vi "_Clear.vi"(6 "Variant in":variant, 8 "error in (no error)":errorcluster, 9 "Shift Pressed?":bool, 10 "QD Combo Box Ref":refnum<vi>, 11 "QD Launch VI Ref":refnum<vi>) -> (0 "error out":errorcluster, 4 "Variant out":variant)   [LabVIEW 2014, in "NEVSTOP QD Shortcuts.lvlib"]
uses:
  NEVSTOP QD Shortcuts.lvlib
panel:
  # "Do not change the connector pane of this VI.\n\nSee the block diagram for directions on how to use this template."
  # "Specify the name of the Undo transaction"
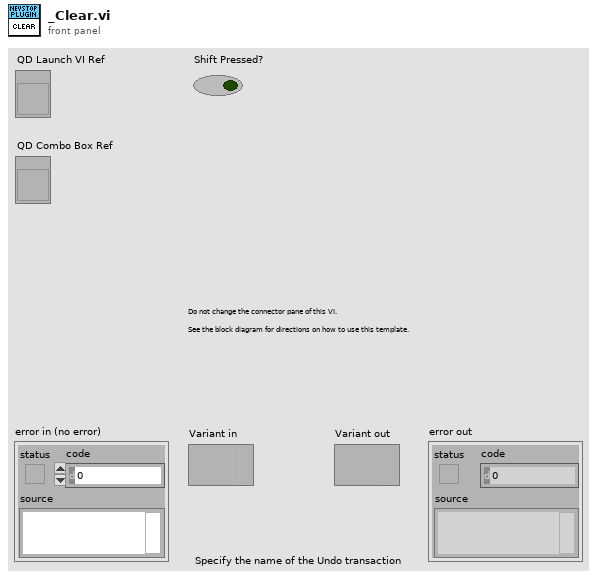
[diagram p1: front panel]
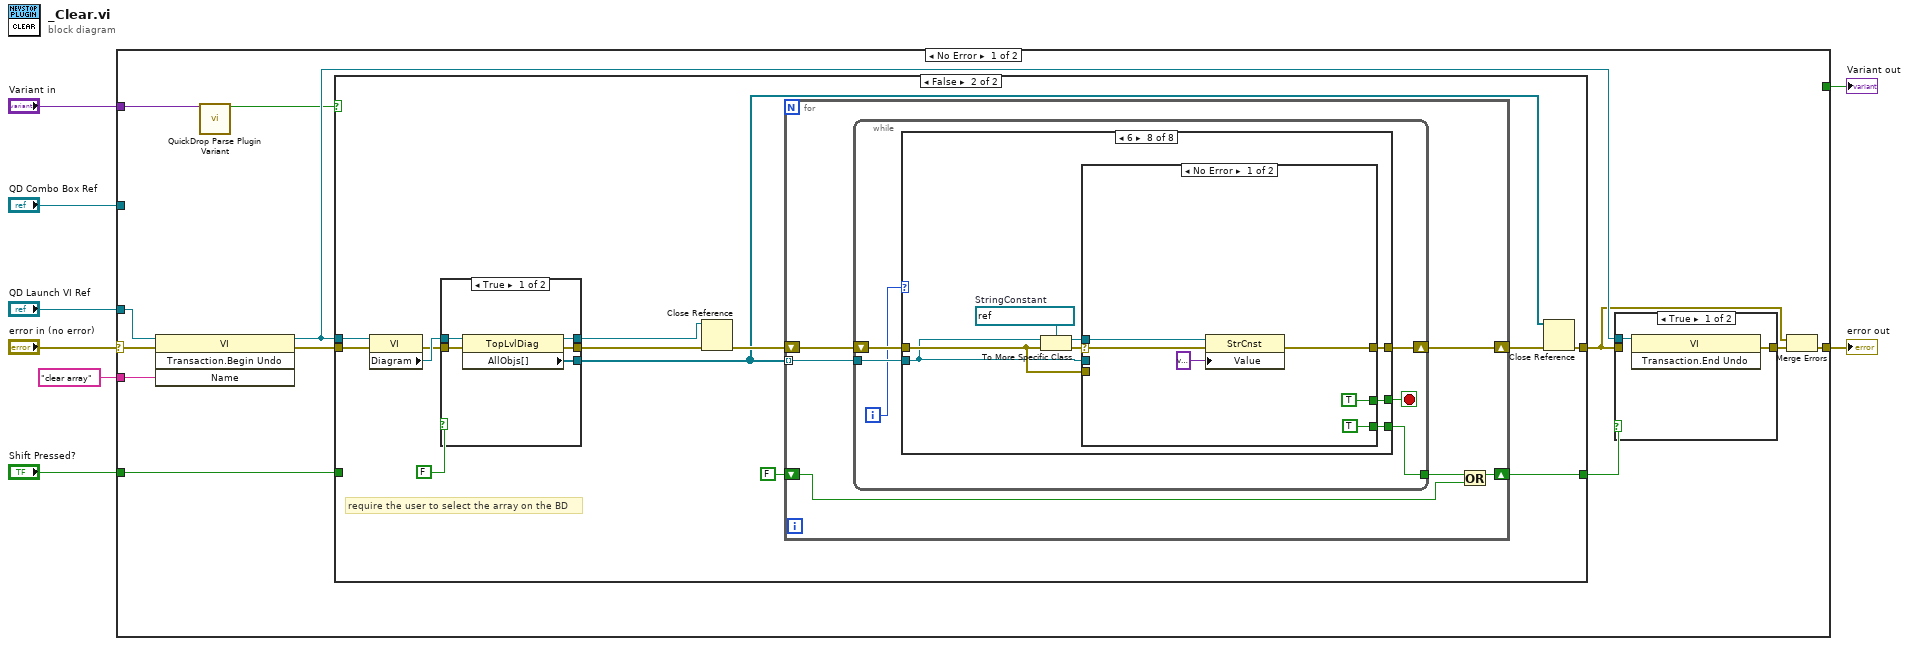
[diagram p0: block diagram]
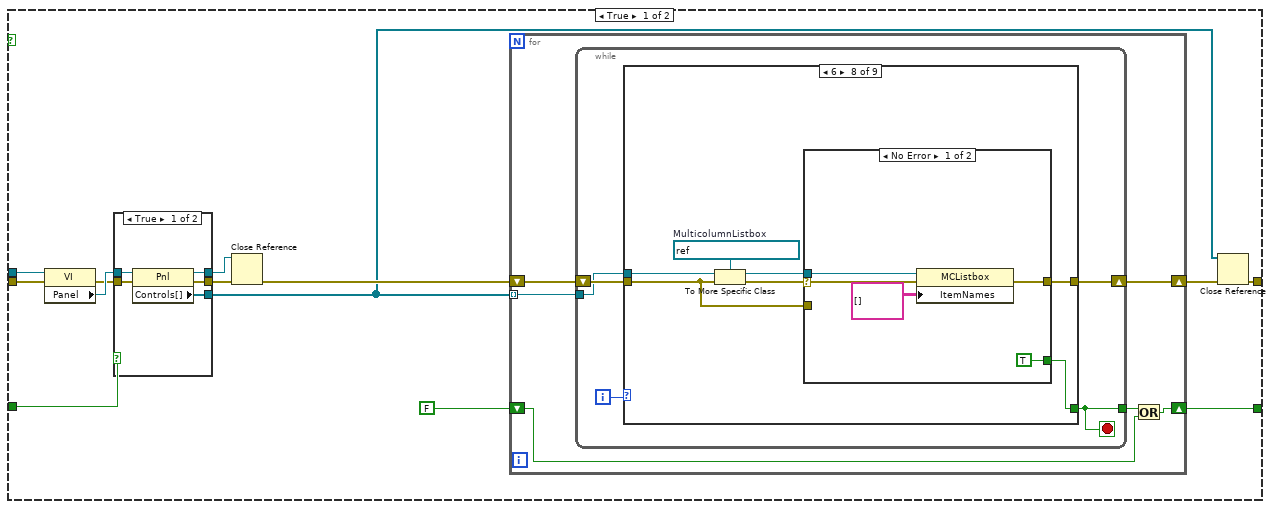
[diagram p2: hidden frame]
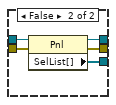
[diagram p3: hidden frame]
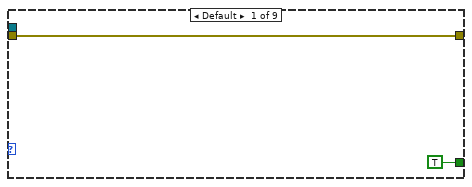
[diagram p4: hidden frame]
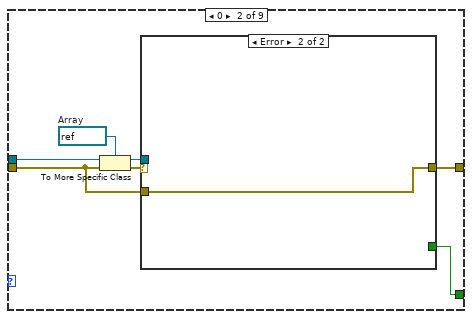
[diagram p5: hidden frame]
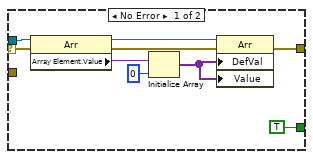
[diagram p6: hidden frame]
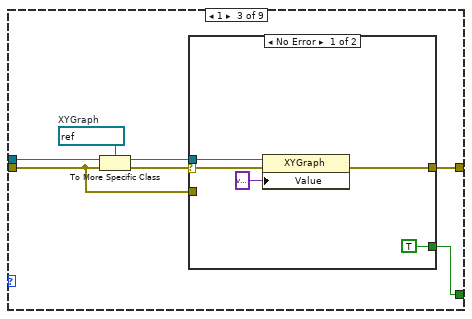
[diagram p7: hidden frame]
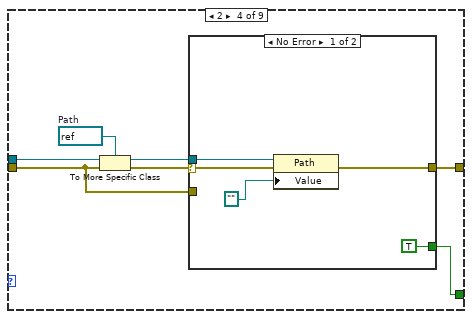
[diagram p9: hidden frame]
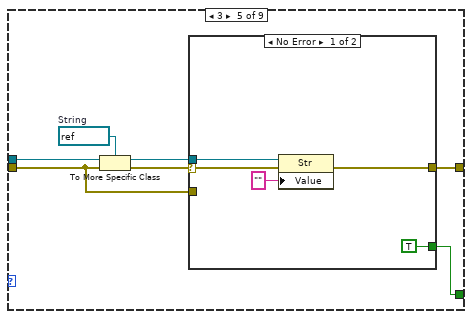
[diagram p11: hidden frame]
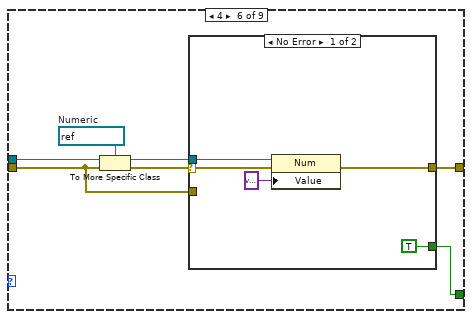
[diagram p13: hidden frame]
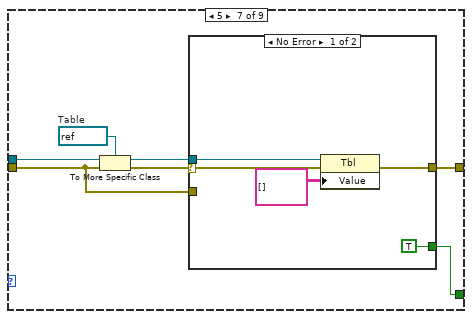
[diagram p15: hidden frame]
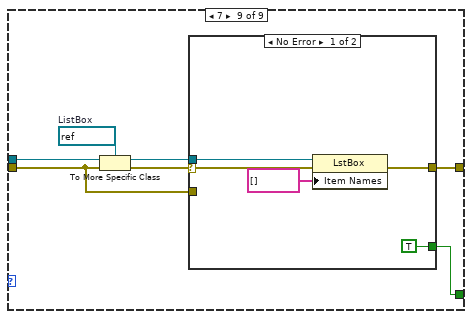
[diagram p18: hidden frame]
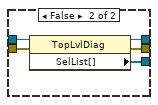
[diagram p20: hidden frame]
diagram:
  n1 = case shown="No Error" "error in (no error)" {
    selector: "error in (no error)" -> [w20 w316]
    tunnel: [w10 w316] -> w7
    tunnel: "QD Launch VI Ref" -> [w19 _]
    tunnel: "Shift Pressed?" -> [w14 _]
    tunnel: "QD Combo Box Ref" -> [_ _]
    tunnel: "Variant in" -> [w21 _]
    tunnel: "clear array" ("Undo Name") -> [w18 _]
    tunnel: [TRUE _] -> w1
    frame No Error {
      n2 = invoke class="VI" method="Transaction.Begin Undo"(reference=w19, error in=w20, "Name"=w18) -> (reference out=w13:refnum<vi>, error out=w16:errorcluster)  [unwired: 1 in, 2 out]
      n3 = call <vilib>:"QuickDrop Parse Plugin Variant.vi"("QDKS Variant in"=w21) -> ("QD Launch VI Panel?"=w12:bool)  [unwired: 12 in, 2 out]
      n4 = case shown="False" w12 {
        tunnel: w16 -> [w34 w178]
        tunnel: [w30 w175] -> w9
        tunnel: w14 -> [w25 _]
        tunnel: w13 -> [w28 w173]
        tunnel: [w23 w169] -> w11
        frame True {
          n5 = property class="VI"(reference=w28, error in=w34) -> (error out=w26:errorcluster, "Panel"=w27:refnum<vi>)  [unwired: 1 out]
          n6 = case shown="True" w25 {
            tunnel: [w39 w44] -> w32
            tunnel: [w38 w43] -> w31
            tunnel: [w37 w42] -> w29
            tunnel: w27 -> [w36 w41]
            tunnel: w26 -> [w35 w40]
            frame True {
              n7 = property class="Pnl"(reference=w36, error in=w35) -> (reference out=w38:refnum<vi>, error out=w39:errorcluster, "Controls[]"=w37:refnum<vi>[])
            }
            frame False {
              n8 = property class="Pnl"(reference=w41, error in=w40) -> (reference out=w43:refnum<vi>, error out=w44:errorcluster, "SelList[]"=w42:refnum<vi>[])
            }
          }
          n9 = Close Reference(reference=w31, error in (no error)=w32) -> (error out=w33:errorcluster)
          n10 = for {
            shift-right: [w50] -> w24
            shift-left: w33 -> [w49]
            tunnel: w29 -> [w48] mode=indexing
            shift-right: [w46] -> w23
            shift-left: FALSE -> [w45]
            n11 = while {
              tunnel: w48 -> [w53]
              tunnel: [w52] -> w47
              shift-right: [w55] -> w50
              shift-left: w49 -> [w54]
              i -> [w51]
              stop <- w52 stop-if-true
              n12 = case shown="6" w51 {
                tunnel: [w57 w64 w81 w94 w107 w120 w133 w146 w159] -> w55
                tunnel: w54 -> [w57 w61 w78 w91 w104 w117 w130 w143 w156]
                tunnel: w53 -> [_ w60 w77 w90 w103 w116 w129 w142 w155]
                tunnel: [TRUE w58 w75 w88 w101 w114 w127 w140 w153] -> w52
                frame Default {
                }
                frame 0 {
                  w59 = refnum<vi> refnum  # Array
                  n13 = To More Specific Class(target class=w59, reference=w60, error in=w61) -> (specific class reference=w63:refnum<vi>, error out=w62:errorcluster)
                  n14 = case shown="Error" w62 {
                    selector: w62 -> [w68 _]
                    tunnel: [w67 w74] -> w64
                    tunnel: w63 -> [w69 _]
                    tunnel: w61 -> [_ w74]
                    tunnel: [TRUE _] -> w58
                    frame No Error {
                      n15 = property class="Arr"(reference=w69, error in=w68) -> (reference out=w72:refnum<vi>, error out=w73:errorcluster, "Array Element.Value"=w71:variant)
                      n16 = Initialize Array(w71, 0 ("dimension size")) -> (w66:variant[])
                      n17 = property class="Arr"(reference=w72, error in=w73, "DefVal"=w66, "Value"=w66) -> (error out=w67:errorcluster)  [unwired: 1 out]
                    }
                    frame Error {
                    }
                  }
                }
                frame 1 {
                  w76 = refnum<vi> refnum  # XYGraph
                  n18 = To More Specific Class(target class=w76, reference=w77, error in=w78) -> (specific class reference=w80:refnum<vi>, error out=w79:errorcluster)
                  n19 = case shown="No Error" w79 {
                    selector: w79 -> [w86 _]
                    tunnel: [w84 w87] -> w81
                    tunnel: w80 -> [w85 _]
                    tunnel: w78 -> [_ w87]
                    tunnel: [TRUE _] -> w75
                    frame No Error {
                      n20 = property class="XYGraph"(reference=w85, error in=w86, "Value"=variant) -> (error out=w84:errorcluster)  [unwired: 1 out]
                    }
                    frame Error {
                    }
                  }
                }
                frame 2 {
                  w89 = refnum<vi> refnum  # Path
                  n21 = To More Specific Class(target class=w89, reference=w90, error in=w91) -> (specific class reference=w93:refnum<vi>, error out=w92:errorcluster)
                  n22 = case shown="No Error" w92 {
                    selector: w92 -> [w99 _]
                    tunnel: [w97 w100] -> w94
                    tunnel: w93 -> [w98 _]
                    tunnel: w91 -> [_ w100]
                    tunnel: [TRUE _] -> w88
                    frame No Error {
                      n23 = property class="Path"(reference=w98, error in=w99, "Value"=path "") -> (error out=w97:errorcluster)  [unwired: 1 out]
                    }
                    frame Error {
                    }
                  }
                }
                frame 3 {
                  w102 = refnum<vi> refnum  # String
                  n24 = To More Specific Class(target class=w102, reference=w103, error in=w104) -> (specific class reference=w106:refnum<vi>, error out=w105:errorcluster)
                  n25 = case shown="No Error" w105 {
                    selector: w105 -> [w112 _]
                    tunnel: [w110 w113] -> w107
                    tunnel: w106 -> [w111 _]
                    tunnel: w104 -> [_ w113]
                    tunnel: [TRUE _] -> w101
                    frame No Error {
                      n26 = property class="Str"(reference=w111, error in=w112, "Value"="") -> (error out=w110:errorcluster)  [unwired: 1 out]
                    }
                    frame Error {
                    }
                  }
                }
                frame 4 {
                  w115 = refnum<vi> refnum  # Numeric
                  n27 = To More Specific Class(target class=w115, reference=w116, error in=w117) -> (specific class reference=w119:refnum<vi>, error out=w118:errorcluster)
                  n28 = case shown="No Error" w118 {
                    selector: w118 -> [w125 _]
                    tunnel: [w123 w126] -> w120
                    tunnel: w119 -> [w124 _]
                    tunnel: w117 -> [_ w126]
                    tunnel: [TRUE _] -> w114
                    frame No Error {
                      n29 = property class="Num"(reference=w124, error in=w125, "Value"=variant) -> (error out=w123:errorcluster)  [unwired: 1 out]
                    }
                    frame Error {
                    }
                  }
                }
                frame 5 {
                  w128 = refnum<vi> refnum  # Table
                  n30 = To More Specific Class(target class=w128, reference=w129, error in=w130) -> (specific class reference=w132:refnum<vi>, error out=w131:errorcluster)
                  n31 = case shown="No Error" w131 {
                    selector: w131 -> [w138 _]
                    tunnel: [w136 w139] -> w133
                    tunnel: w132 -> [w137 _]
                    tunnel: w130 -> [_ w139]
                    tunnel: [TRUE _] -> w127
                    frame No Error {
                      n32 = property class="Tbl"(reference=w137, error in=w138, "Value"=string[][] []) -> (error out=w136:errorcluster)  [unwired: 1 out]
                    }
                    frame Error {
                    }
                  }
                }
                frame 6 {
                  w141 = refnum<vi> refnum  # MulticolumnListbox
                  n33 = To More Specific Class(target class=w141, reference=w142, error in=w143) -> (specific class reference=w145:refnum<vi>, error out=w144:errorcluster)
                  n34 = case shown="No Error" w144 {
                    selector: w144 -> [w151 _]
                    tunnel: [w149 w152] -> w146
                    tunnel: w145 -> [w150 _]
                    tunnel: w143 -> [_ w152]
                    tunnel: [TRUE _] -> w140
                    frame No Error {
                      n35 = property class="MCListbox"(reference=w150, error in=w151, "ItemNames"=string[][] [] ("Item Names")) -> (error out=w149:errorcluster)  [unwired: 1 out]
                    }
                    frame Error {
                    }
                  }
                }
                frame 7 {
                  w154 = refnum<vi> refnum  # ListBox
                  n36 = To More Specific Class(target class=w154, reference=w155, error in=w156) -> (specific class reference=w158:refnum<vi>, error out=w157:errorcluster)
                  n37 = case shown="No Error" w157 {
                    selector: w157 -> [w164 _]
                    tunnel: [w162 w165] -> w159
                    tunnel: w158 -> [w163 _]
                    tunnel: w156 -> [_ w165]
                    tunnel: [TRUE _] -> w153
                    frame No Error {
                      n38 = property class="LstBox"(reference=w163, error in=w164, "Item Names"=string[] []) -> (error out=w162:errorcluster)  [unwired: 1 out]
                    }
                    frame Error {
                    }
                  }
                }
              }
            }
            n39 = Or(x=w47, y=w45) -> (x .or. y?=w46:bool)
          }
          n40 = Close Reference(reference=w29, error in (no error)=w24) -> (error out=w30:errorcluster)
        }
        frame False {
          # "require the user to select the array on the BD"
          n41 = property class="VI"(reference=w173, error in=w178) -> (error out=w171:errorcluster, "Diagram"=w172:refnum<vi>)  [unwired: 1 out]
          n42 = case shown="True" FALSE {
            tunnel: [w183 w188] -> w176
            tunnel: [w182 w187] -> w166
            tunnel: [w181 w186] -> w174
            tunnel: w172 -> [w180 w185]
            tunnel: w171 -> [w179 w184]
            frame True {
              n43 = property class="TopLvlDiag"(reference=w180, error in=w179) -> (reference out=w182:refnum<vi>, error out=w183:errorcluster, "AllObjs[]"=w181:refnum<vi>[])
            }
            frame False {
              n44 = property class="TopLvlDiag"(reference=w185, error in=w184) -> (reference out=w187:refnum<vi>, error out=w188:errorcluster, "SelList[]"=w186:refnum<vi>[])
            }
          }
          n45 = Close Reference(reference=w166, error in (no error)=w176) -> (error out=w177:errorcluster)
          n46 = for {
            shift-right: [w194] -> w170
            shift-left: w177 -> [w193]
            tunnel: w174 -> [w189] mode=indexing
            shift-right: [w191] -> w169
            shift-left: FALSE -> [w190]
            n47 = while {
              tunnel: [w198] -> w192
              tunnel: w189 -> [w197]
              shift-right: [w200] -> w194
              shift-left: w193 -> [w199]
              i -> [w196]
              stop <- w195 stop-if-true
              n48 = case shown="6" w196 {
                tunnel: [w202 w210 w229 w244 w259 w274 w289 w304] -> w200
                tunnel: w199 -> [w202 w207 w226 w241 w256 w271 w286 w301]
                tunnel: [_ w205 w224 w239 w254 w269 w284 w299] -> w198
                tunnel: w197 -> [_ w204 w223 w238 w253 w268 w283 w298]
                tunnel: [TRUE w203 w222 w237 w252 w267 w282 w297] -> w195
                frame Default {
                }
                frame 0 {
                  w206 = refnum<vi> refnum  # ArrayConstant
                  n49 = To More Specific Class(target class=w206, reference=w204, error in=w207) -> (specific class reference=w209:refnum<vi>, error out=w208:errorcluster)
                  n50 = case shown="No Error" w208 {
                    selector: w208 -> [w215 _]
                    tunnel: [w214 w221] -> w210
                    tunnel: w209 -> [w216 _]
                    tunnel: w207 -> [_ w221]
                    tunnel: [TRUE _] -> w205
                    tunnel: w204 -> [_ _]
                    tunnel: [TRUE _] -> w203
                    frame No Error {
                      n51 = property class="ArrCnst"(reference=w216, error in=w215) -> (reference out=w219:refnum<vi>, error out=w220:errorcluster, "Element.Value"=w218:variant)
                      n52 = Initialize Array(w218, 0 ("dimension size")) -> (w212:variant[])
                      n53 = property class="ArrCnst"(reference=w219, error in=w220, "Value"=w212) -> (error out=w214:errorcluster)  [unwired: 1 out]
                    }
                    frame Error {
                    }
                  }
                }
                frame 1 {
                  w225 = refnum<vi> refnum  # NumericConstant
                  n54 = To More Specific Class(target class=w225, reference=w223, error in=w226) -> (specific class reference=w228:refnum<vi>, error out=w227:errorcluster)
                  n55 = case shown="No Error" w227 {
                    selector: w227 -> [w235 _]
                    tunnel: [w233 w236] -> w229
                    tunnel: w228 -> [w234 _]
                    tunnel: w226 -> [_ w236]
                    tunnel: [TRUE _] -> w224
                    tunnel: w223 -> [_ _]
                    tunnel: [TRUE _] -> w222
                    frame No Error {
                      n56 = property class="NumericConstant"(reference=w234, error in=w235, "Value"=variant) -> (error out=w233:errorcluster)  [unwired: 1 out]
                    }
                    frame Error {
                    }
                  }
                }
                frame 2 {
                  w240 = refnum<vi> refnum  # Table
                  n57 = To More Specific Class(target class=w240, reference=w238, error in=w241) -> (specific class reference=w243:refnum<vi>, error out=w242:errorcluster)
                  n58 = case shown="No Error" w242 {
                    selector: w242 -> [w250 _]
                    tunnel: [w248 w251] -> w244
                    tunnel: w243 -> [w249 _]
                    tunnel: w241 -> [_ w251]
                    tunnel: [TRUE _] -> w239
                    tunnel: w238 -> [_ _]
                    tunnel: [TRUE _] -> w237
                    frame No Error {
                      n59 = property class="Tbl"(reference=w249, error in=w250, "Value"=string[][] []) -> (error out=w248:errorcluster)  [unwired: 1 out]
                    }
                    frame Error {
                    }
                  }
                }
                frame 3 {
                  w255 = refnum<vi> refnum  # MulticolumnListbox
                  n60 = To More Specific Class(target class=w255, reference=w253, error in=w256) -> (specific class reference=w258:refnum<vi>, error out=w257:errorcluster)
                  n61 = case shown="No Error" w257 {
                    selector: w257 -> [w265 _]
                    tunnel: [w263 w266] -> w259
                    tunnel: w258 -> [w264 _]
                    tunnel: w256 -> [_ w266]
                    tunnel: [TRUE _] -> w254
                    tunnel: w253 -> [_ _]
                    tunnel: [TRUE _] -> w252
                    frame No Error {
                      n62 = property class="MCListbox"(reference=w264, error in=w265, "ItemNames"=string[][] [] ("Item Names")) -> (error out=w263:errorcluster)  [unwired: 1 out]
                    }
                    frame Error {
                    }
                  }
                }
                frame 4 {
                  w270 = refnum<vi> refnum  # ListBox
                  n63 = To More Specific Class(target class=w270, reference=w268, error in=w271) -> (specific class reference=w273:refnum<vi>, error out=w272:errorcluster)
                  n64 = case shown="No Error" w272 {
                    selector: w272 -> [w280 _]
                    tunnel: [w278 w281] -> w274
                    tunnel: w273 -> [w279 _]
                    tunnel: w271 -> [_ w281]
                    tunnel: [TRUE _] -> w269
                    tunnel: w268 -> [_ _]
                    tunnel: [TRUE _] -> w267
                    frame No Error {
                      n65 = property class="LstBox"(reference=w279, error in=w280, "Item Names"=string[] []) -> (error out=w278:errorcluster)  [unwired: 1 out]
                    }
                    frame Error {
                    }
                  }
                }
                frame 5 {
                  w285 = refnum<vi> refnum  # PathConstant
                  n66 = To More Specific Class(target class=w285, reference=w283, error in=w286) -> (specific class reference=w288:refnum<vi>, error out=w287:errorcluster)
                  n67 = case shown="No Error" w287 {
                    selector: w287 -> [w295 _]
                    tunnel: [w293 w296] -> w289
                    tunnel: w288 -> [w294 _]
                    tunnel: w286 -> [_ w296]
                    tunnel: [TRUE _] -> w284
                    tunnel: w283 -> [_ _]
                    tunnel: [TRUE _] -> w282
                    frame No Error {
                      n68 = property class="PthCnst"(reference=w294, error in=w295, "Value"=variant) -> (error out=w293:errorcluster)  [unwired: 1 out]
                    }
                    frame Error {
                    }
                  }
                }
                frame 6 {
                  w300 = refnum<vi> refnum  # StringConstant
                  n69 = To More Specific Class(target class=w300, reference=w298, error in=w301) -> (specific class reference=w303:refnum<vi>, error out=w302:errorcluster)
                  n70 = case shown="No Error" w302 {
                    selector: w302 -> [w310 _]
                    tunnel: [w308 w311] -> w304
                    tunnel: w303 -> [w309 _]
                    tunnel: w301 -> [_ w311]
                    tunnel: [TRUE _] -> w299
                    tunnel: w298 -> [_ _]
                    tunnel: [TRUE _] -> w297
                    frame No Error {
                      n71 = property class="StrCnst"(reference=w309, error in=w310, "Value"=variant) -> (error out=w308:errorcluster)  [unwired: 1 out]
                    }
                    frame Error {
                    }
                  }
                }
              }
            }
            n72 = Or(x=w192, y=w190) -> (x .or. y?=w191:bool)
          }
          n73 = Close Reference(reference=w174, error in (no error)=w170) -> (error out=w175:errorcluster)
        }
      }
      n74 = case shown="True" w11 {
        tunnel: w13 -> [w312 w314]
        tunnel: [w313 w315] -> w15
        tunnel: w9 -> [_ _]
        frame True {
          n75 = invoke class="VI" method="Transaction.End Undo"(reference=w312) -> (error out=w313:errorcluster)  [unwired: 2 in, 2 out]
        }
        frame False {
          n76 = invoke class="VI" method="Transaction.Fail"(reference=w314) -> (error out=w315:errorcluster)  [unwired: 2 in, 2 out]
        }
      }
      n77 = Merge Errors(w9, w15) -> (w10:errorcluster)
    }
    frame Error {
    }
  }
  "error out" <- w7
  "Variant out" <- w1
